vi "Process.vi"(8 "error in":errorcluster, 11 "PolyA":refnum<class "PolyA.lvclass">) -> (0 "error out":errorcluster, 3 "PolyA out":refnum<class "PolyA.lvclass">)   [LabVIEW 2014, in "PolyA.lvclass"]
doc: "JKI State Machine Objects (SMO) 1.4.0.57\nJKI - JKI\nCopyright (c) 2018, JKI"
uses:
  PolyA.lvclass
  <vilib>/JKI/JKI SMO/SMO/Typedefs/Parent Call--Enum.ctl
  Query Payload -- cluster.ctl
  PolyA.lvclass/PolyA.ctl
  <vilib>/Analysis/polynomials.llb/Scalar Polynomial Evaluation (DBL).vi
  <vilib>/JKI/JKI SMO/SMO/SMO.lvclass
  <vilib>/Analysis/NI_AALPro.lvlib
panel:
  # "For instructions on how to use the JKI State Machine Objects, examples and video tutorials, visit:\nhttp://jki.net/state-machine-objects/\n\nJKI State Machine Objects™\nhttp://jki.net/state-machine-objects/\nCopyright (C) 2005-2015, JKI <info@jki.net>\nALL RIGHTS RESERVED"
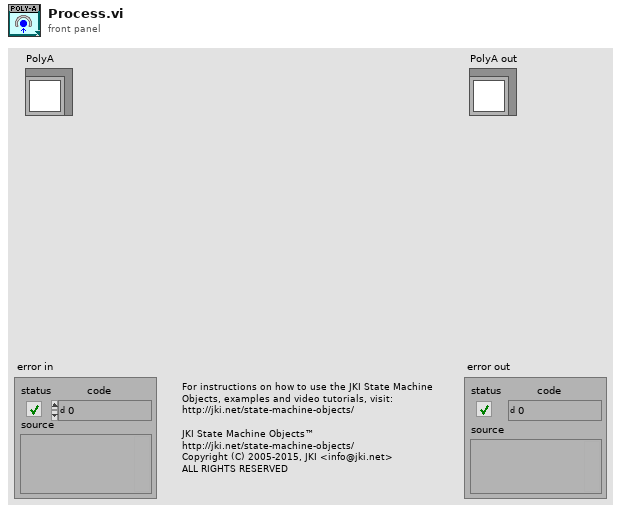
[diagram p1: front panel]
types:
  T1 = typedef "SMO.lvclass/Parent Call--Enum.ctl" = enum16{"Allows parent to run", "Does not request parent to run"}
  T2 = typedef "PolyA.lvclass/Query Payload -- cluster.ctl" = cluster{"value":dbl, "notifier":refnum<notifier>}
  T3 = enum32{"invalid app kind", "Development System", "Run Time System", "Student Edition", "Embedded LabVIEW", "Evaluation", "Custom"}
  T4 = enum32{"Invalid", "Standard", "Closed", "Hidden", "Minimized", "Maximized"}
  T5 = cluster{"Core":cluster{"Current VI Reference":refnum<vi>, "Close Panel on Exit?":bool, "error":errorcluster}, "Self Reference":refnum<class "PolyA.lvclass">, "Polynomials":dbl[], "queue":refnum<queue>}
  T6 = cluster{"Current VI Reference":refnum<vi>, "Close Panel on Exit?":bool, "error":errorcluster}
  T7 = typedef "SMO.lvclass/Protected Events.ctl" = cluster{"StopProcesses":refnum<user-event>, "AbortProcesses":refnum<user-event>, "Config Changed":refnum<user-event>, "Dependency":refnum<user-event>}
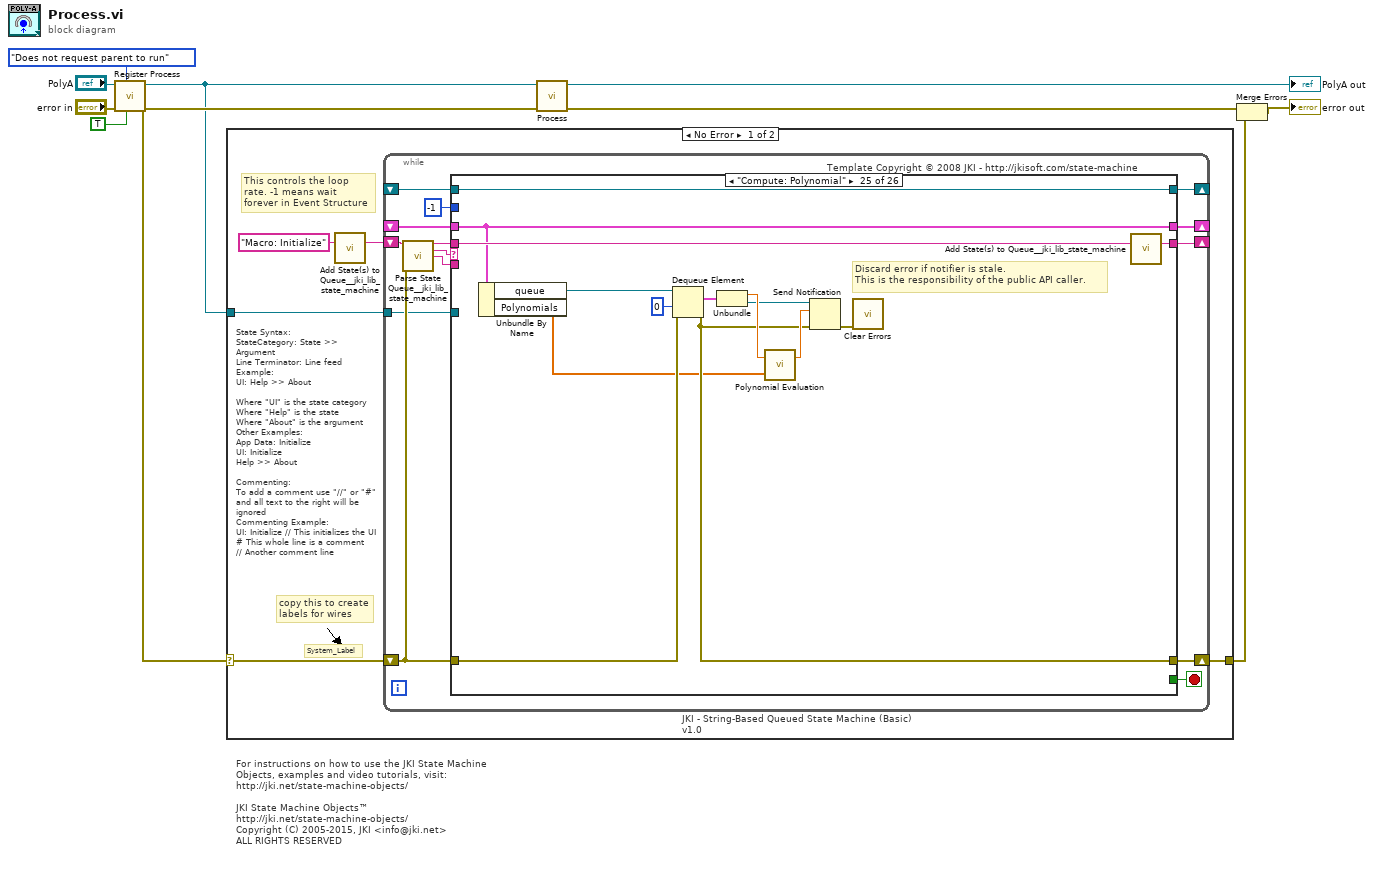
[diagram p0: block diagram]
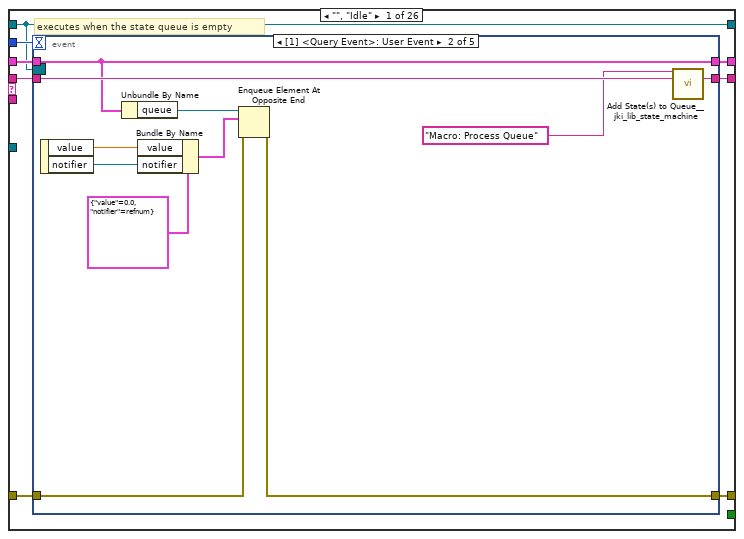
[diagram p2: hidden frame]
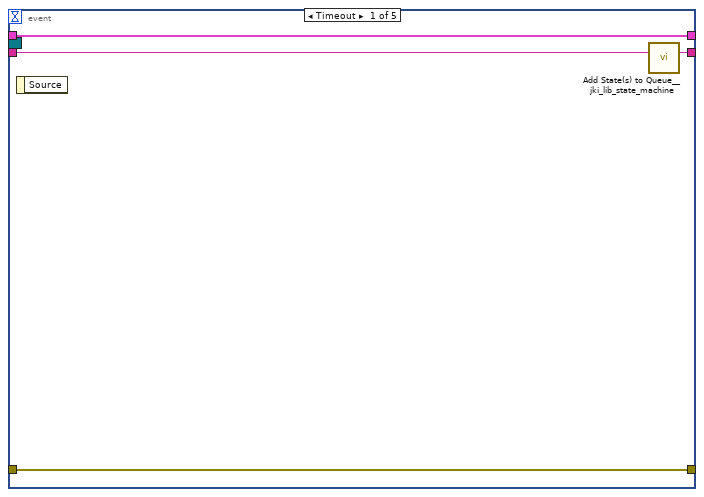
[diagram p3: hidden frame]
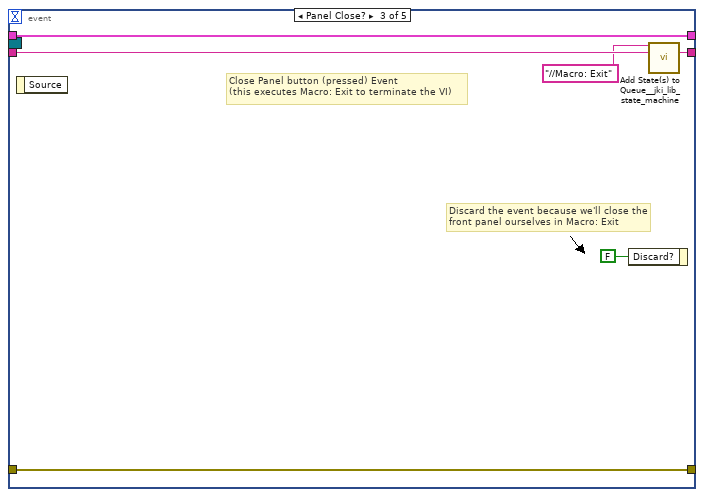
[diagram p4: hidden frame]
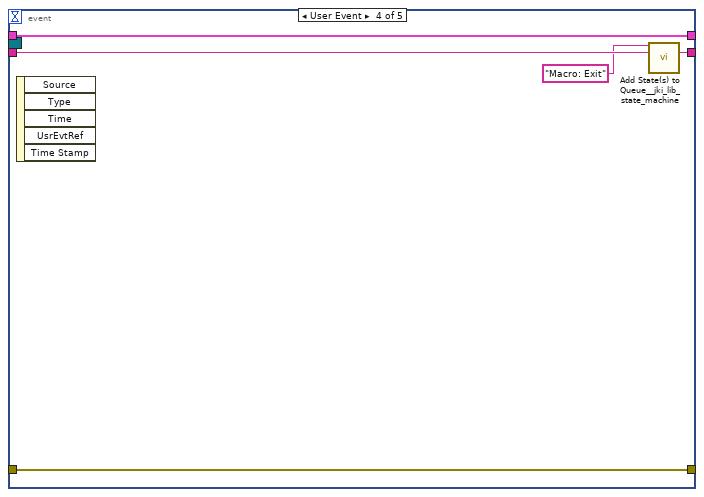
[diagram p5: hidden frame]
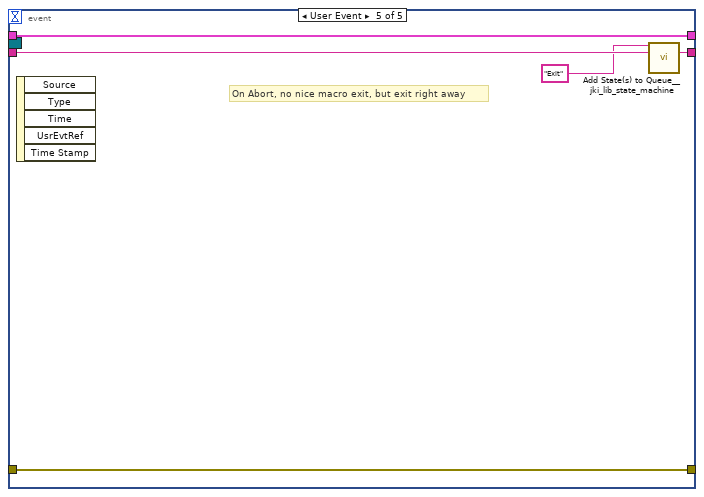
[diagram p6: hidden frame]
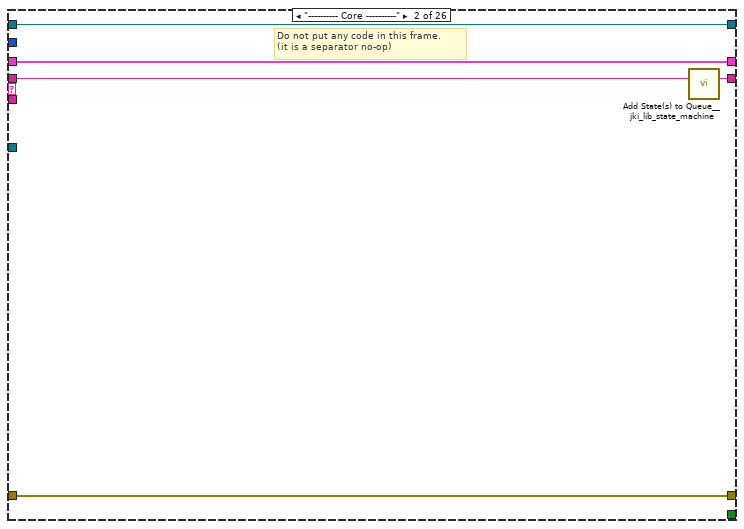
[diagram p7: hidden frame]
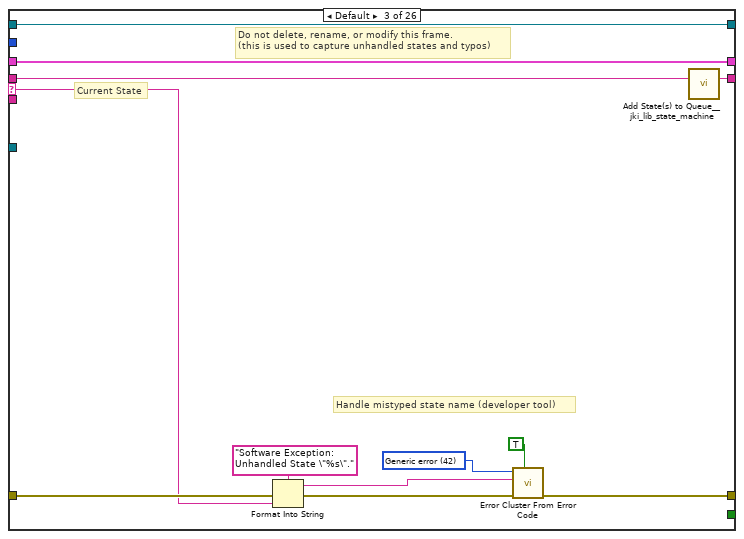
[diagram p8: hidden frame]
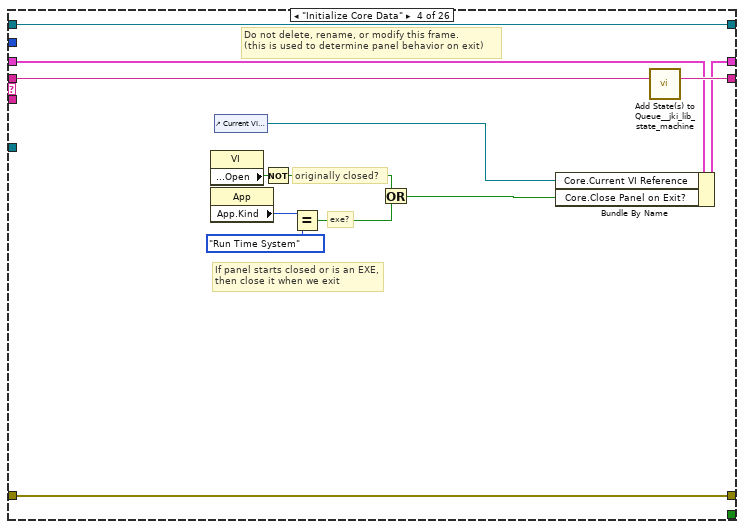
[diagram p9: hidden frame]
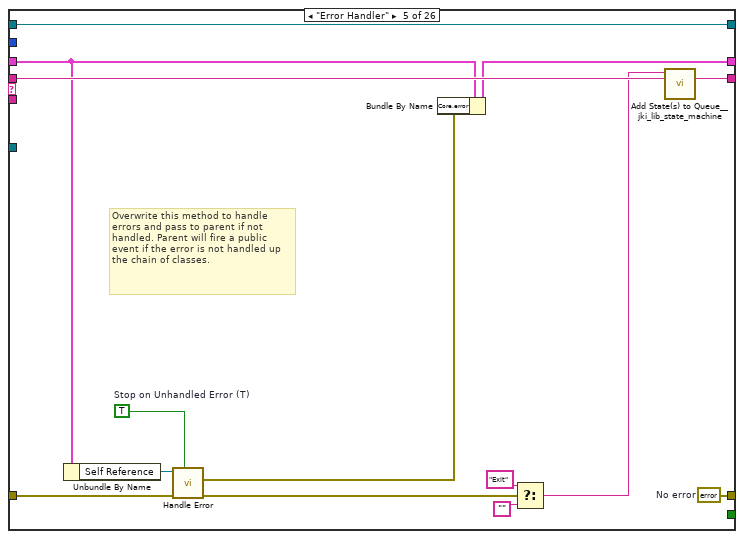
[diagram p10: hidden frame]
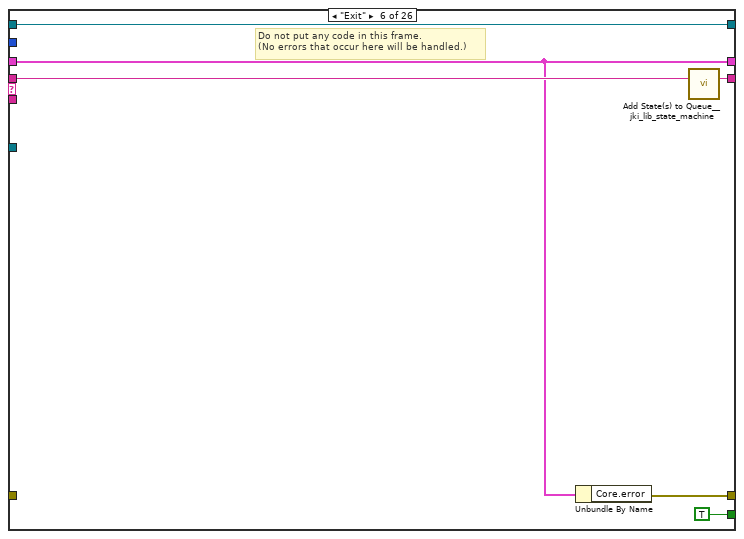
[diagram p11: hidden frame]
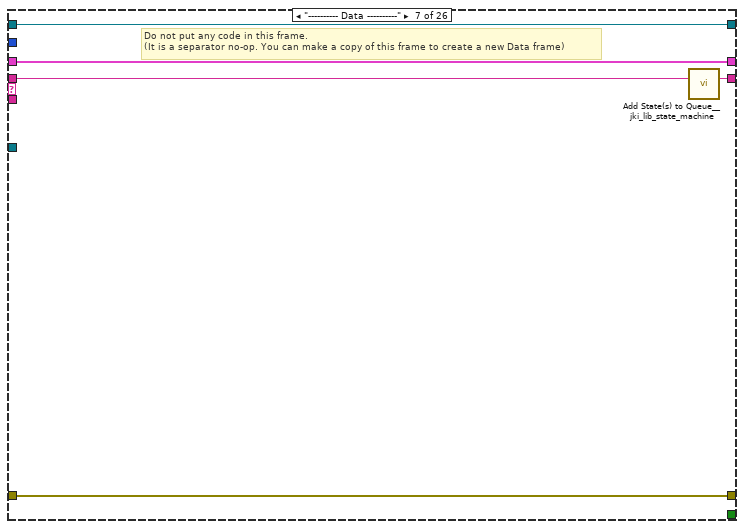
[diagram p12: hidden frame]
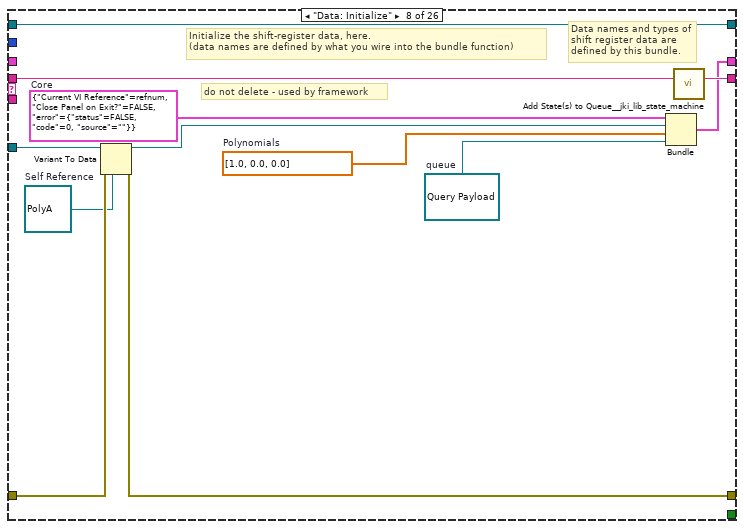
[diagram p13: hidden frame]
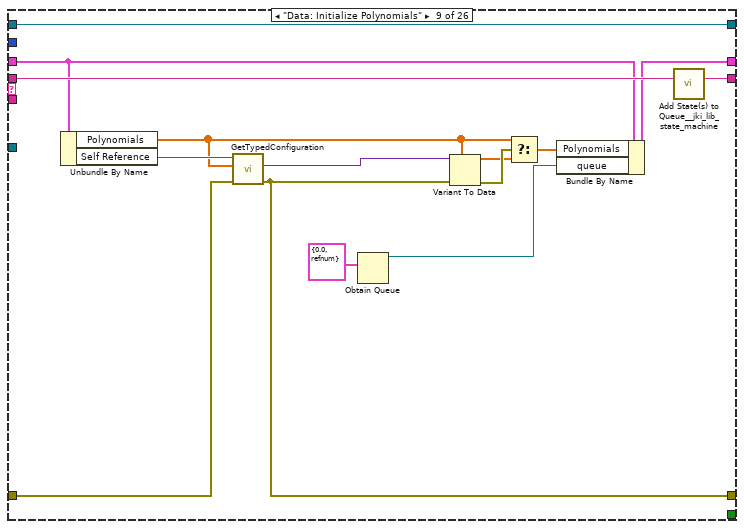
[diagram p14: hidden frame]
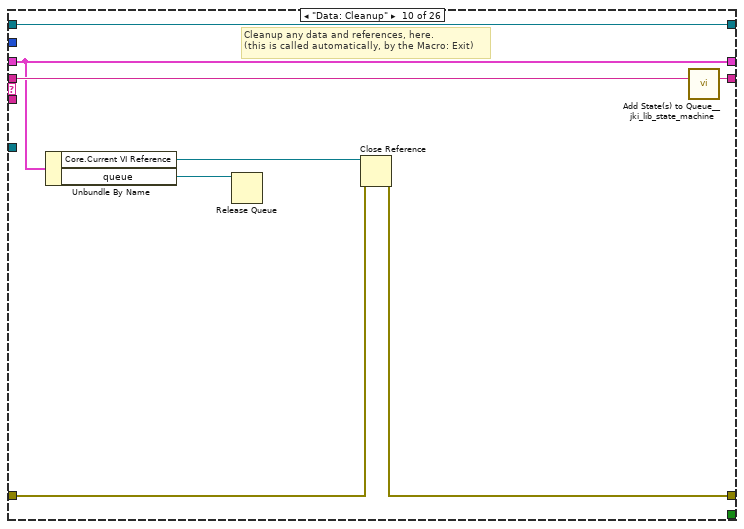
[diagram p15: hidden frame]
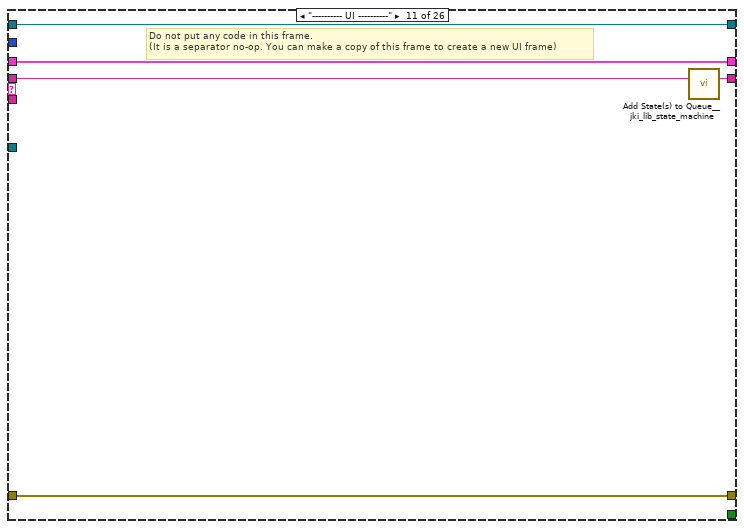
[diagram p16: hidden frame]
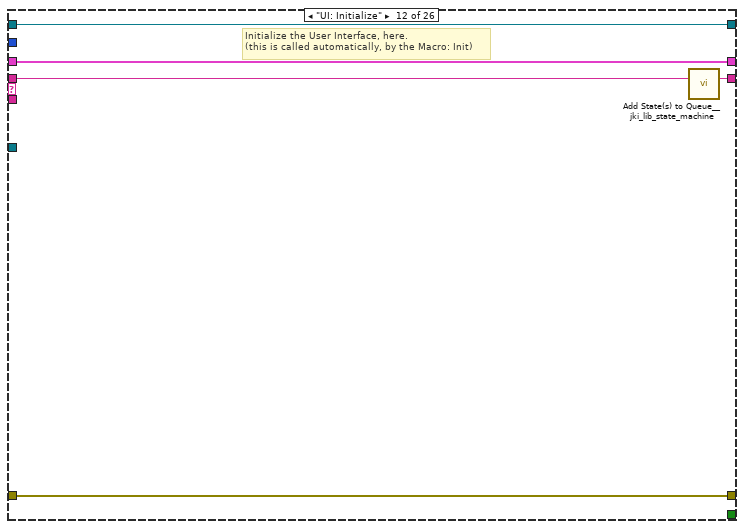
[diagram p17: hidden frame]
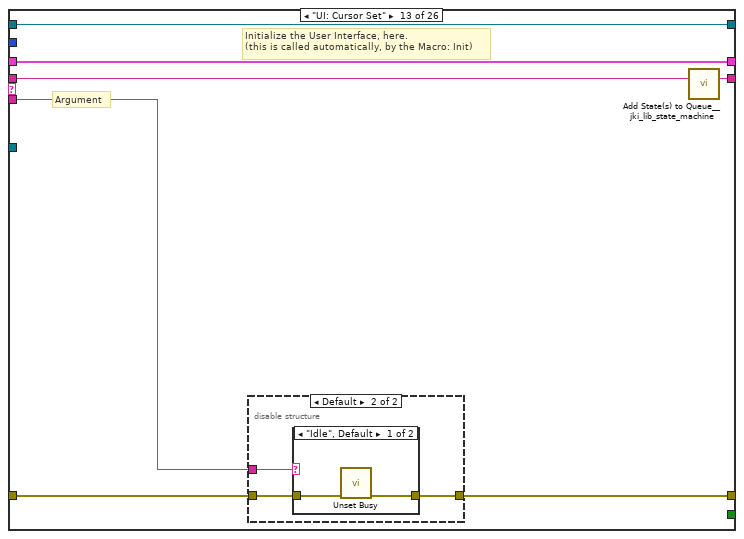
[diagram p18: hidden frame]
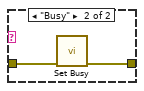
[diagram p20: hidden frame]
diagram:
  # "For instructions on how to use the JKI State Machine Objects, examples and video tutorials, visit:\nhttp://jki.net/state-machine-objects/\n\nJKI State Machine Objects™\nhttp://jki.net/state-machine-objects/\nCopyright (C) 2005-2015, JKI <info@jki.net>\nALL RIGHTS RESERVED"
  n1 = call <vilib>:"Register Process.vi"("Forces Self to Run (F)"=TRUE, "Parent Call"=Parent_Call--Enum."Does not request parent to run", "error in (no error)"="error in", "SMO"="PolyA") -> ("error out"=w10:errorcluster, "SMO out"=w9:refnum<class "PolyA.lvclass">)  [unwired: 6 in]
  n2 = case shown="No Error" w10 {
    selector: w10 -> [w12 w321]
    tunnel: w9 -> [w13 _]
    tunnel: [w11 w321] -> w7
    frame No Error {
      # "State Syntax:\nStateCategory: State >> Argument\nLine Terminator: Line feed\nExample:\nUI: Help >> About\n\nWhere \"UI\" is the state category\nWhere \"Help\" is the state\nWhere \"About\" is the argument\nOther Examples:\nApp Data: Initialize\nUI: Initialize\nHelp >> About\n\nCommenting:\nTo add a comment use \"//\" or \"#\" and all text to the right will be ignored\nCommenting Example:\nUI: Initialize // This initializes the UI\n# This whole line is a comment\n// Another comment line"
      # "copy this to create labels for wires"
      # "This controls the loop rate. -1 means wait forever in Event Structure"
      # "System_Label"
      n3 = call <vilib>:"Add State(s) to Queue__jki_lib_state_machine.vi"("State(s) in (\"\")"="Macro: Initialize") -> ("States Out"=w15:string)  [unwired: 14 in]
      n4 = while "JKI - String-Based Queued State Machine (Basic) v1.0" {
        shift-right: [w22] -> _
        shift-left: _ -> [w21]
        shift-right: [w25] -> w11
        shift-left: w12 -> [w19]
        shift-right: [w24] -> _
        shift-left: w15 -> [w26]
        tunnel: w13 -> [w18]
        shift-right: [w17] -> _
        shift-left: _ -> [w16]
        stop <- w23 stop-if-true
        # "Template Copyright © 2008 JKI - http://jkisoft.com/state-machine"
        n5 = call <vilib>:"Parse State Queue__jki_lib_state_machine.vi"("State Queue"=w26, "Error In (no error)"=w19) -> ("Remaining States"=w28:string, "Current State"=w29:string, "Arguments"=w27:string)  [unwired: 11 in]
        n6 = case shown="\"Compute: Polynomial\"" w29 {
          selector: w29 -> [_ _ w75 _ _ _ _ _ _ _ _ _ _ _ _ _ _ _ _ _ _ _ _ _ _ _]
          tunnel: w28 -> [w37 w73 w79 w98 w112 w118 w123 w135 w150 w158 w163 w168 w175 w191 w223 w232 w238 w252 w257 w268 w273 w284 w290 w295 w309 w320]
          tunnel: w27 -> [_ _ _ _ _ _ _ _ _ _ _ _ w169 w185 _ _ _ _ _ _ _ _ _ _ _ _]
          tunnel: w21 -> [w35 w70 w77 w89 w106 w114 w120 _ w147 w153 w160 w166 w173 w187 w220 w228 w234 w243 w254 w265 w270 w282 w288 w293 w300 w310]
          tunnel: [w34 w71 w81 w95 w107 w113 w121 w131 w138 w154 w161 w165 w170 w188 w221 w230 w236 w250 w255 w259 w271 w279 w286 w291 w299 w317] -> w25
          tunnel: w19 -> [w33 w71 w80 w95 w108 _ w121 w132 w139 w155 w161 w165 w171 w189 w221 w230 w236 w250 w255 w260 w271 w280 w286 w291 w304 w317]
          tunnel: [w36 w72 w78 w97 w111 w117 w122 w134 w149 w157 w162 w167 w174 w190 w222 w231 w237 w251 w256 w267 w272 w283 w289 w294 w308 w319] -> w24
          tunnel: [_ _ _ _ _ TRUE _ _ _ _ _ _ _ _ _ _ _ _ _ _ _ _ _ _ _ _] -> w23
          tunnel: [w32 w70 w77 w96 w105 w114 w120 w133 w146 w153 w160 w166 w173 w187 w220 w228 w234 w243 w254 w265 w270 w282 w288 w293 w300 w310] -> w22
          tunnel: -1 ("Timeout") -> [w31 _ _ _ _ _ _ _ _ _ _ _ _ _ _ _ _ _ _ _ _ _ _ _ _ _]
          tunnel: w18 -> [_ _ _ _ _ _ _ w130 _ _ _ _ _ _ _ _ _ _ _ _ _ _ _ _ _ _]
          tunnel: [w30 w69 w74 w86 w110 w115 w119 w128 w148 w152 w159 w164 w172 w184 w219 w229 w235 w244 w253 w266 w269 w274 w287 w292 w307 w318] -> w17
          tunnel: w16 -> [w30 w69 w74 w86 w110 w115 w119 w128 w148 w152 w159 w164 w172 w184 w219 w229 w235 w244 w253 w266 w269 _ w287 w292 w307 w318]
          frame "", "Idle" {
            # "executes when the state queue is empty"
            n7 = event shown="[1] <Query Event>: User Event" {
              selector: w30 -> [_ _ _ _ _]
              dyn-events: _ -> [_ _ _ _ _]
              timeout: w31 -> [_ _ _ _ _]
              tunnel: w37 -> [w41 w52 w58 w63 w68]
              tunnel: [w40 w51 w57 w62 w67] -> w36
              tunnel: w35 -> [w39 w50 w55 w60 w65]
              tunnel: [w38 w42 w56 w61 w66] -> w34
              tunnel: w33 -> [w38 w43 w56 w61 w66]
              tunnel: [w39 w50 w55 w60 w65] -> w32
              event Timeout {
                n8 = event-data() -> ()  [unwired: 1 in, 1 out]
                n9 = call <vilib>:"Add State(s) to Queue__jki_lib_state_machine.vi"("State(s) in (\"\")"=w41) -> ("States Out"=w40:string)  [unwired: 14 in]
              }
              event User Event {
                n10 = event-data() -> ("value"=w45:dbl, "notifier"=w46:refnum<notifier>)  [unwired: 1 in]
                n11 = Unbundle By Name(w50) -> ("queue"=w49:refnum<queue>)
                n12 = Bundle By Name(cluster=T2 {"value"=0.0, "notifier"=refnum} ("Query Payload"), "value"=w45, "notifier"=w46) -> (w44:T2)
                n13 = Enqueue Element At Opposite End(queue=w49, element=w44, error in (no error)=w43) -> (error out=w42:errorcluster)  [unwired: 1 in, 2 out]
                n14 = call <vilib>:"Add State(s) to Queue__jki_lib_state_machine.vi"("State(s) in Front (\"\")"="Macro: Process Queue" ("t"), "State(s) in (\"\")"=w52) -> ("States Out"=w51:string)  [unwired: 13 in]
              }
              event Panel Close? {
                # "Discard the event because we'll close the front panel ourselves in Macro: Exit"
                # "Close Panel button (pressed) Event\n(this executes Macro: Exit to terminate the VI)"
                n15 = event-data() -> ()  [unwired: 1 in, 1 out]
                n16 = event-data("Discard?"=FALSE) -> ()  [unwired: 1 in, 1 out]
                n17 = call <vilib>:"Add State(s) to Queue__jki_lib_state_machine.vi"("State(s) in Front (\"\")"="//Macro: Exit", "State(s) in (\"\")"=w58) -> ("States Out"=w57:string)  [unwired: 13 in]
              }
              event User Event {
                n18 = event-data() -> ()  [unwired: 1 in, 5 out]
                n19 = call <vilib>:"Add State(s) to Queue__jki_lib_state_machine.vi"("State(s) in Front (\"\")"="Macro: Exit", "State(s) in (\"\")"=w63) -> ("States Out"=w62:string)  [unwired: 13 in]
              }
              event User Event {
                # "On Abort, no nice macro exit, but exit right away"
                n20 = event-data() -> ()  [unwired: 1 in, 5 out]
                n21 = call <vilib>:"Add State(s) to Queue__jki_lib_state_machine.vi"("State(s) in Front (\"\")"="Exit", "State(s) in (\"\")"=w68) -> ("States Out"=w67:string)  [unwired: 13 in]
              }
            }
          }
          frame "---------- Core ----------" {
            # "Do not put any code in this frame.\n(it is a separator no-op)"
            n22 = call <vilib>:"Add State(s) to Queue__jki_lib_state_machine.vi"("State(s) in (\"\")"=w73) -> ("States Out"=w72:string)  [unwired: 14 in]
          }
          frame Default {
            w84 = 42 items=["No error", "Argument error", "Memory is full", "Out of zone", "End of file", "File already open", "Generic file I/O error", "File not found", "File permission error", "Disk is full", "Duplicate path", "Too many files open", "System feature not enabled", "Resource file not found", "Cannot add resource", "Resource not found", "Image not found", "Image memory error", "Pen does not exist", "Config type invalid", "Config token not found", "Config parse error", "Config memory error", "Bad external code format", "Bad external code offset", "External code not present", "Null window", "Destroy window error", "Null menu", "Print aborted", "Bad print record", "Print driver error", "Windows error during printing", "Memory error during printing", "Print dialog error", "Generic print error", "Invalid device refnum", "Device not found", "Device parameter error", "Device unit error", "Cannot open device", "Device call aborted", "Generic error", "Cancelled by user", "Object ID too low", "Object ID too high", "Object not in heap", "Unknown heap", "Unknown object (invalid DefProc)", "Unknown object (DefProc not in table)", "Message out of range", "Invalid (null) method", "Unknown message", "Manager call not supported", "Bad address", "Network operation in progress", "Network operation timed out", "Connection is busy", "Network attribute not supported", "Network error", "Address in use", "System out of memory", "Connection aborted", "Connection refused", "Not connected", "Already connected", "Connection closed", "Initialization error (interapplication manager)", "Bad occurrence", "Wait on unbound occurrence handler", "Occurrence queue overflow", "Datalog type conflict", "Unused", "Unrecognized type (interapplication manager)", "Memory corrupt", "Failed to make temporary DLL", "Old CIN version", "Drag socket not found", "Failed to load drop-object", "Failed to register OLE object", "Failed to release OLE object", "Format specifier type mismatch", "Unknown format specifier", "Too few format specifiers", "Too many format specifiers", "Scan failed", "Newer CIN version", "Error converting to variant", "Runtime menu error", "Password tampered", "Variant attribute not found", "Incompatible variant data type", "Event data is not available", "Event Store is not present", "Occurrence is not found", "Event Queue is not created", "Event info is not available", "Refnum passed is NULL", "Error retrieving Class GUID", "Error retrieving CoClass GUID", "Error retrieving TypeLib GUID.", "Bad built application magic bytes.", "Specific driver is different from the specific driver associated with the Logical Name.", "There is no session opened to the class driver.", "Max Error", "MAX - Error with config objects", "MAX - Error loading configuration", "MAX - Group not supported"]
            # "Current State"
            # "Do not delete, rename, or modify this frame.\n(this is used to capture unhandled states and typos)"
            # "Handle mistyped state name (developer tool)"
            n23 = Format Into String(format string="Software Exception: Unhandled State \"%s\"." ("message"), error in=w80, w75) -> (resulting string=w83:string, error out=w82:errorcluster)  [unwired: 1 in]
            n24 = call <vilib>:"Error Cluster From Error Code.vi"("show call chain? (False)"=TRUE, "error in (no error)"=w82, "error message (\"\")"=w83, "error code (0)"=w84) -> ("error out"=w81:errorcluster)  [unwired: 5 in]
            n25 = call <vilib>:"Add State(s) to Queue__jki_lib_state_machine.vi"("State(s) in (\"\")"=w79) -> ("States Out"=w78:string)  [unwired: 14 in]
          }
          frame "Initialize Core Data" {
            # "Do not delete, rename, or modify this frame.\n(this is used to determine panel behavior on exit)"
            # "originally closed?"
            # "exe?"
            # "If panel starts closed or is an EXE, then close it when we exit"
            n26 = property class="VI"() -> ("Front Panel.Open"=w94:bool)  [unwired: 2 in, 2 out]
            n27 = property class="App"() -> ("App.Kind"=w93:T3)  [unwired: 2 in, 2 out]
            n28 = control-ref of="Current VI Reference"() -> (w87:refnum<vi>)
            n29 = Not(x=w94) -> (.not. x?=w91:bool)
            n30 = Equal?(x=w93, y=T3."Run Time System" ("Application:Kind")) -> (x = y?=w90:bool)
            n31 = Or(x=w91, y=w90) -> (x .or. y?=w88:bool)
            n32 = Bundle By Name(cluster=w89, "Core.Current VI Reference"=w87, "Core.Close Panel on Exit?"=w88) -> (w96:T5)
            n33 = call <vilib>:"Add State(s) to Queue__jki_lib_state_machine.vi"("State(s) in (\"\")"=w98) -> ("States Out"=w97:string)  [unwired: 14 in]
          }
          frame "Error Handler" {
            w99 = TRUE  # Stop on Unhandled Error (T)
            w107 = errorcluster {"status"=FALSE, "code"=0, "source"=""}  # No error
            # "Overwrite this method to handle errors and pass to parent if not handled. Parent will fire a public event if the error is not handled up the chain of classes."
            n34 = Unbundle By Name(w106) -> ("Self Reference"=w109:refnum<class "PolyA.lvclass">)
            n35 = call-dynamic "Handle Error.vi"("Stop on Unhandled Error (T)"=w99, "error in"=w108, "SMO"=w109) -> ("handling error"=w100:errorcluster, "Unhandled error"=w103:errorcluster)  [unwired: 6 in, 1 out]
            n36 = Bundle By Name(cluster=w106, "Core.error"=w103) -> (w105:T5)
            n37 = Select(t="Exit", s=w100, f="") -> (s? t:f=w104:string)
            n38 = call <vilib>:"Add State(s) to Queue__jki_lib_state_machine.vi"("State(s) in Front (\"\")"=w104, "State(s) in (\"\")"=w112) -> ("States Out"=w111:string)  [unwired: 13 in]
          }
          frame "Exit" {
            # "Do not put any code in this frame.\n(No errors that occur here will be handled.)"
            n39 = Unbundle By Name(w114) -> ("Core.error"=w113:errorcluster)
            n40 = call <vilib>:"Add State(s) to Queue__jki_lib_state_machine.vi"("State(s) in (\"\")"=w118) -> ("States Out"=w117:string)  [unwired: 14 in]
          }
          frame "---------- Data ----------" {
            # "Do not put any code in this frame.\n(It is a separator no-op. You can make a copy of this frame to create a new Data frame)"
            n41 = call <vilib>:"Add State(s) to Queue__jki_lib_state_machine.vi"("State(s) in (\"\")"=w123) -> ("States Out"=w122:string)  [unwired: 14 in]
          }
          frame "Data: Initialize" {
            w124 = refnum<queue> refnum  # queue
            w125 = dbl[] [1.0, 0.0, 0.0]  # Polynomials
            w126 = refnum<class "PolyA.lvclass"> refnum  # Self Reference
            w127 = T6 {"Current VI Reference"=refnum, "Close Panel on Exit?"=FALSE, "error"={"status"=FALSE, "code"=0, "source"=""}}  # Core
            # "do not delete - used by framework"
            # "Data names and types of shift register data are defined by this bundle."
            # "Initialize the shift-register data, here.\n(data names are defined by what you wire into the bundle function)"
            n42 = Variant To Data(error in=w132, type=w126, Variant=w130) -> (data=w129:refnum<class "PolyA.lvclass">, error out=w131:errorcluster)
            n43 = Bundle("Core"=w127, "Self Reference"=w129, "Polynomials"=w125, "queue"=w124) -> (w133:T5)  [unwired: 1 in]
            n44 = call <vilib>:"Add State(s) to Queue__jki_lib_state_machine.vi"("State(s) in (\"\")"=w135) -> ("States Out"=w134:string)  [unwired: 14 in]
          }
          frame "Data: Initialize Polynomials" {
            n45 = Unbundle By Name(w147) -> ("Polynomials"=w141:dbl[], "Self Reference"=w142:refnum<class "PolyA.lvclass">)
            n46 = call <vilib>:"GetTypedConfiguration.vi"("error in (no error)"=w139, "Default value"=w141, "SMO"=w142) -> ("error out"=w138:errorcluster, "Variant"=w140:variant)  [unwired: 4 in, 3 out]
            n47 = Obtain Queue(element data type=T2 {"value"=0.0, "notifier"=refnum} ("Query Payload")) -> (queue out=w137:refnum<queue>)  [unwired: 4 in, 2 out]
            n48 = Variant To Data(error in=w138, type=w141, Variant=w140) -> (data=w144:dbl[], error out=w145:errorcluster)
            n49 = Select(t=w141, s=w145, f=w144) -> (s? t:f=w143:dbl[])
            n50 = Bundle By Name(cluster=w147, "Polynomials"=w143, "queue"=w137) -> (w146:T5)
            n51 = call <vilib>:"Add State(s) to Queue__jki_lib_state_machine.vi"("State(s) in (\"\")"=w150) -> ("States Out"=w149:string)  [unwired: 14 in]
          }
          frame "Data: Cleanup" {
            # "Cleanup any data and references, here.\n(this is called automatically, by the Macro: Exit)"
            n52 = Unbundle By Name(w153) -> ("Core.Current VI Reference"=w156:refnum<vi>, "queue"=w151:refnum<queue>)
            n53 = Release Queue(queue=w151) -> ()  [unwired: 2 in, 3 out]
            n54 = Close Reference(reference=w156, error in (no error)=w155) -> (error out=w154:errorcluster)
            n55 = call <vilib>:"Add State(s) to Queue__jki_lib_state_machine.vi"("State(s) in (\"\")"=w158) -> ("States Out"=w157:string)  [unwired: 14 in]
          }
          frame "---------- UI ----------" {
            # "Do not put any code in this frame.\n(It is a separator no-op. You can make a copy of this frame to create a new UI frame)"
            n56 = call <vilib>:"Add State(s) to Queue__jki_lib_state_machine.vi"("State(s) in (\"\")"=w163) -> ("States Out"=w162:string)  [unwired: 14 in]
          }
          frame "UI: Initialize" {
            # "Initialize the User Interface, here.\n(this is called automatically, by the Macro: Init)"
            n57 = call <vilib>:"Add State(s) to Queue__jki_lib_state_machine.vi"("State(s) in (\"\")"=w168) -> ("States Out"=w167:string)  [unwired: 14 in]
          }
          frame "UI: Cursor Set" {
            # "Argument"
            # "Initialize the User Interface, here.\n(this is called automatically, by the Macro: Init)"
            n58 = disable-structure shown="Default" {
              disable-tunnel: w171 -> [w176 w179]
              disable-tunnel: [w176 w178] -> w170
              disable-tunnel: w169 -> [_ w177]
              frame condition #0 {
              }
              frame condition #1 (active) {
                n59 = case shown="\"Idle\", Default" w177 {
                  tunnel: w179 -> [w181 w183]
                  tunnel: [w180 w182] -> w178
                  frame "Idle", Default {
                    n60 = call <vilib>:"Unset Busy.vi"("error in (no error)"=w181) -> ("error out"=w180:errorcluster)  [unwired: 10 in]
                  }
                  frame "Busy" {
                    n61 = call <vilib>:"Set Busy.vi"("error in (no error)"=w183) -> ("error out"=w182:errorcluster)  [unwired: 9 in, 1 out]
                  }
                }
              }
            }
            n62 = call <vilib>:"Add State(s) to Queue__jki_lib_state_machine.vi"("State(s) in (\"\")"=w175) -> ("States Out"=w174:string)  [unwired: 14 in]
          }
          frame "UI: Front Panel State" {
            # "Argument"
            # "Set Front Panel Open or Closed\n(Usage: \"UI: Front Panel State >> Open|Close\")"
            n63 = Unbundle By Name(w187) -> ("Core.Current VI Reference"=w186:refnum<vi>)
            n64 = disable-structure shown="Default" {
              disable-tunnel: w189 -> [w195 w218]
              disable-tunnel: [w194 w218] -> w188
              disable-tunnel: w186 -> [w193 _]
              disable-tunnel: w185 -> [w192 _]
              frame condition #0 (active) {
                n65 = case shown="\"Close\"" w192 {
                  tunnel: w195 -> [w199 w212]
                  tunnel: [w201 w213] -> w194
                  tunnel: w193 -> [w200 w210]
                  frame "Open", Default {
                    n66 = property class="VI"(reference=w200, error in=w199) -> (reference out=w197:refnum<vi>, error out=w198:errorcluster, "FP.State"=w196:T4)
                    n67 = case shown="\"Closed\"" w196 {
                      tunnel: [w204 w207] -> w201
                      tunnel: w198 -> [w203 w207]
                      tunnel: w197 -> [w202 _]
                      frame "Closed" {
                        n68 = invoke class="VI" method="FP.Open"(reference=w202, error in=w203, "Activate"=TRUE, "State"=T4."Standard") -> (error out=w204:errorcluster)  [unwired: 1 in, 4 out]
                      }
                      frame Default {
                      }
                    }
                  }
                  frame "Close" {
                    n69 = property class="VI"(reference=w210, error in=w212) -> (reference out=w209:refnum<vi>, error out=w211:errorcluster, "FP.State"=w208:T4)
                    n70 = case shown="Default" w208 {
                      tunnel: [w214 w217] -> w213
                      tunnel: w211 -> [w214 w216]
                      tunnel: w209 -> [_ w215]
                      frame "Invalid", "Closed" {
                      }
                      frame Default {
                        n71 = invoke class="VI" method="FP.Close"(reference=w215, error in=w216) -> (error out=w217:errorcluster)  [unwired: 1 in, 2 out]
                      }
                    }
                  }
                }
              }
              frame condition #1 {
              }
            }
            n72 = call <vilib>:"Add State(s) to Queue__jki_lib_state_machine.vi"("State(s) in (\"\")"=w191) -> ("States Out"=w190:string)  [unwired: 14 in]
          }
          frame "---------- Macro ----------" {
            # "Do not put any code in this frame.\n(It is a separator no-op. You can make a copy of this frame to create a new Macro frame)"
            n73 = call <vilib>:"Add State(s) to Queue__jki_lib_state_machine.vi"("State(s) in (\"\")"=w223) -> ("States Out"=w222:string)  [unwired: 14 in]
          }
          frame "Macro: Initialize" {
            w226 = "//UI: Initialize\n//UI: Front Panel State >> Open"  # //UI: Initialize //UI: Front Panel State >> Open
            # "Initialization Macro\n(This is called once, when the VI starts)"
            n74 = call <vilib>:"Add State(s) to Queue__jki_lib_state_machine.vi"("State(s) in Front (\"\")"="Data: Initialize\nInitialize Core Data\nEvents: Register\nData: Initialize Polynomials", "State(s) in (\"\")"="Process: Sync", "State(s) at Back (\"\")"=w226) -> ("States Out"=w225:string)  [unwired: 12 in]
            n75 = call <vilib>:"Add State(s) to Queue__jki_lib_state_machine.vi"("State(s) in Front (\"\")"=w225, "State(s) in (\"\")"=w232) -> ("States Out"=w231:string)  [unwired: 13 in]
          }
          frame "Macro: Process Queue" {
            n76 = call <vilib>:"Add State(s) to Queue__jki_lib_state_machine.vi"("State(s) in Front (\"\")"="Compute: Polynomial\nCompute: Check Queue", "State(s) in (\"\")"=w238) -> ("States Out"=w237:string)  [unwired: 13 in]
          }
          frame "Macro: Exit" {
            # "Exit Macro\n(This is called once, when the VI exits)"
            n77 = Unbundle By Name(w243) -> ("Core.Close Panel on Exit?"=w249:bool)
            n78 = Select(t="UI: Front Panel State >> Close", s=w249, f="") -> (s? t:f=w246:string)
            n79 = call <vilib>:"Add State(s) to Queue__jki_lib_state_machine.vi"("State(s) in Front (\"\")"="Data: Cleanup\nEvents: Unregister", "State(s) in (\"\")"="Process: Sync", "State(s) at Back (\"\")"="Exit") -> ("States Out"=w240:string)  [unwired: 12 in]
            n80 = call <vilib>:"Add State(s) to Queue__jki_lib_state_machine.vi"("State(s) in (\"\")"=w246, "State(s) at Back (\"\")"=w240) -> ("States Out"=w245:string)  [unwired: 13 in]
            n81 = call <vilib>:"Add State(s) to Queue__jki_lib_state_machine.vi"("State(s) in Front (\"\")"=w245, "State(s) in (\"\")"=w252) -> ("States Out"=w251:string)  [unwired: 13 in]
          }
          frame "---------- Process ----------" {
            # "Template Separator\n(You can make a copy of, or modify, this frame)"
            n82 = call <vilib>:"Add State(s) to Queue__jki_lib_state_machine.vi"("State(s) in (\"\")"=w257) -> ("States Out"=w256:string)  [unwired: 14 in]
          }
          frame "Process: Sync" {
            n83 = Unbundle By Name(w265) -> ("Self Reference"=w261:refnum<class "PolyA.lvclass">)
            n84 = call <vilib>:"WaitOnProcessSync.vi"("error in (no error)"=w260, "SMO"=w261) -> ("error out"=w259:errorcluster, "Don't run?"=w264:bool)  [unwired: 7 in, 1 out]
            n85 = Select(t="Data: Cleanup\nEvents: Unregister\nExit", s=w264, f="") -> (s? t:f=w258:string)
            n86 = call <vilib>:"Add State(s) to Queue__jki_lib_state_machine.vi"("State(s) in Front (\"\")"=w258, "State(s) in (\"\")"=w268) -> ("States Out"=w267:string)  [unwired: 13 in]
          }
          frame "---------- Events ----------" {
            # "Template Separator\n(You can make a copy of, or modify, this frame)"
            n87 = call <vilib>:"Add State(s) to Queue__jki_lib_state_machine.vi"("State(s) in (\"\")"=w273) -> ("States Out"=w272:string)  [unwired: 14 in]
          }
          frame "Events: Register" {
            # "Expand to add\nmore events"
            n88 = Unbundle By Name(w282) -> ("Self Reference"=w276:refnum<class "PolyA.lvclass">)
            n89 = call <vilib>:"GetProtectedEvents.vi"("SMO"=w276) -> ("error out"=w277:errorcluster, "SMO Protected Events"=w281:T7)  [unwired: 8 in, 1 out]
            n90 = Unbundle By Name(w276) -> ("Query Event"=w275:refnum<user-event>)
            n91 = register-events(w281, w275) -> (reference out=w274:refnum<event-registration>, error out=w278:errorcluster)  [unwired: 2 in]
            n92 = Merge Errors(w280, w278, w277) -> (w279:errorcluster)
            n93 = call <vilib>:"Add State(s) to Queue__jki_lib_state_machine.vi"("State(s) in (\"\")"=w284) -> ("States Out"=w283:string)  [unwired: 14 in]
          }
          frame "Events: Unregister" {
            n94 = Unregister For Events(event registration refnum=w287, error in=w286) -> (error out=w285:errorcluster)
            n95 = call <vilib>:"Clear Errors.vi"("error in (no error)"=w285) -> ()  [unwired: 5 in, 2 out]
            n96 = call <vilib>:"Add State(s) to Queue__jki_lib_state_machine.vi"("State(s) in (\"\")"=w290) -> ("States Out"=w289:string)  [unwired: 14 in]
          }
          frame "---------- Compute ----------" {
            n97 = call <vilib>:"Add State(s) to Queue__jki_lib_state_machine.vi"("State(s) in (\"\")"=w295) -> ("States Out"=w294:string)  [unwired: 14 in]
          }
          frame "Compute: Polynomial" {
            # "Discard error if notifier is stale.\nThis is the responsibility of the public API caller."
            n98 = Unbundle By Name(w300) -> ("queue"=w297:refnum<queue>, "Polynomials"=w296:dbl[])
            n99 = Dequeue Element(queue=w297, timeout in ms (-1)=0, error in (no error)=w304) -> (element=w298:T2, error out=w299:errorcluster)  [unwired: 2 out]
            n100 = Unbundle(w298) -> ("value"=w306:dbl, "notifier"=w303:refnum<notifier>)
            n101 = call-poly <vilib>:"Polynomial Evaluation.vi"("P(x)"=w296, "a"=w306) -> ("P(a)"=w302:dbl)  [unwired: 1 out]
            n102 = Send Notification(notification=w302, notifier=w303, error in (no error)=w299) -> (error out=w301:errorcluster)  [unwired: 1 out]
            n103 = call <vilib>:"Clear Errors.vi"("error in (no error)"=w301) -> ()  [unwired: 5 in, 2 out]
            n104 = call <vilib>:"Add State(s) to Queue__jki_lib_state_machine.vi"("State(s) in (\"\")"=w309) -> ("States Out"=w308:string)  [unwired: 14 in]
          }
          frame "Compute: Check Queue" {
            n105 = Unbundle By Name(w310) -> ("queue"=w316:refnum<queue>)
            n106 = Get Queue Status(queue=w316) -> (# pending remove=w315:i32)  [unwired: 2 in, 7 out]
            n107 = Not Equal To 0?(x=w315) -> (x != 0?=w314:bool)
            n108 = Select(t="Macro: Process Queue", s=w314, f="") -> (s? t:f=w313:string)
            n109 = call <vilib>:"Add State(s) to Queue__jki_lib_state_machine.vi"("State(s) in Front (\"\")"=w313, "State(s) in (\"\")"=w320) -> ("States Out"=w319:string)  [unwired: 13 in]
          }
        }
      }
    }
    frame Error {
    }
  }
  n110 = call-parent "Process.vi"("error in"=w10, "SMO"=w9) -> ("error out"=w8:errorcluster, "SMO out"=→"PolyA out":refnum<class "PolyA.lvclass">)  [unwired: 8 in]
  n111 = Merge Errors(w8, w7) -> (→"error out":errorcluster)
